vi "config-AUXI.vi"(11 "DO List":string[](array[string])) -> ()   [LabVIEW 2024]
uses:
  controls/type.aux.ctl
  <vilib>/Utility/miscctls.llb/LVPointTypeDef.ctl
  controls/typeEnv.ctl
  controls/UiProcHeader.ctl
  <vilib>/Utility/error.llb/Clear Errors.vi
  globals/globals-engine.vi
  <vilib>/Utility/libraryn.llb/Create Directory Recursive.vi
panel:
  in  "Cluster":T1={"Source"="Source ...", "SourceStatus"=FALSE, "Dest"="Auxiliary ...", "DestStatus"=FALSE, "Pulse"=0, "Period"=0, "Proc Name"=""} {"Period" format="Period [s]: %d"; "Pulse" format="Pulse [s]: %d"}
  in  "index":i8=1 min=1 max=10 step=1
  out "deleted path":path
  in  "Menu":cluster{"load":bool, "save":bool}
  in  "Aux Conf":T1[](array[typedef]) {"Period" format="Period [s]: %d"; "Pulse" format="Pulse [s]: %d"}
  in  "DataChanged?":bool=TRUE
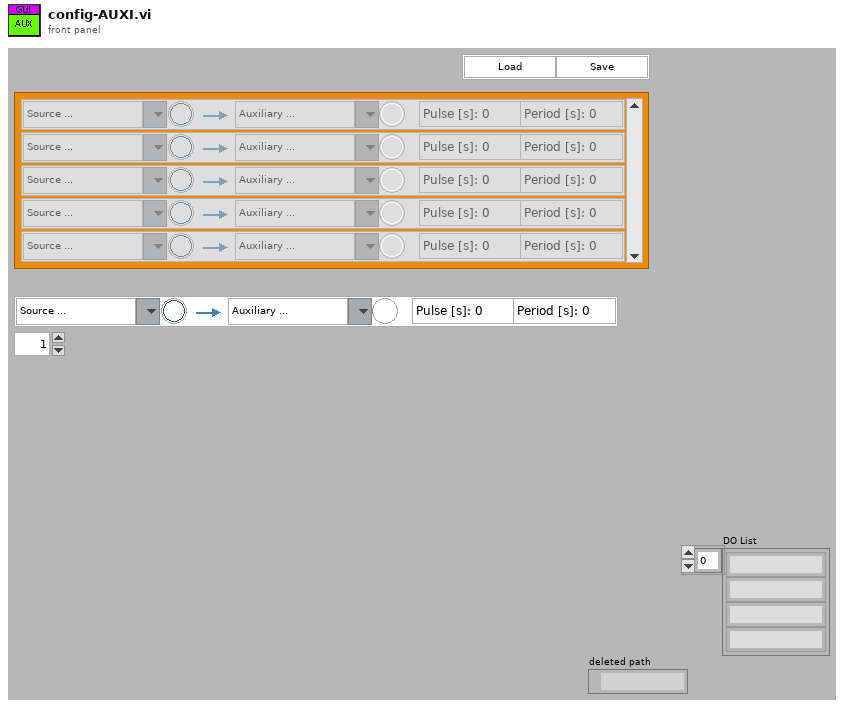
[diagram p1: front panel]
types:
  T1 = typedef "type.aux.ctl" = cluster{"Source":string, "SourceStatus":bool, "Dest":string, "DestStatus":bool, "Pulse":u16, "Period":u16, "Proc Name":string}
  T2 = typedef "typeEnv.ctl" = enum16{"ENV.PRODUCTION", "ENV.TEST.NO-HW", "ENV.TEST.SINGLE-01", "ENV.TEST.SINGLE-02", "ENV.TEST.SINGLE-02 AI 0", "ENV.TEST.SINGLE-03"}
  T3 = typedef "LVPointTypeDef.ctl" = cluster{"Horizontal":i16, "Vertical":i16}
  T4 = typedef "UiProcHeader.ctl" = cluster{"Procedure Name":string, "Running":bool, "tags":string}
  T5 = typedef "UiStepBuilder.ctl" = cluster{"Step Function":T6, "ParamString":string, "Step Label":string}
  T6 = typedef "type.step-builder.ctl" = enum16{"NO_OPERATION", "DELAY-JUMP", "DELAY", "JUMP", "COMPLETE", "SCHEDULER", "IRR-CHECK", "UNIT-CHECK", "UNIT-SAMPLE", "UNIT-DOSE", "LOG-REPORT", "LOG-MESSAGE", "IO-READ", "IO-READ-MANY", "IO-WRITE", "IO-COMPARE-OUT", "IO-COMPARE-IN", "PROC-START", "PROC-STOP", "PROC-LOAD", "PROC-IS-COMPLETED", "RECORD-MOVE", "GET-RH", "GET-UV", "GET-WD", "GET-WS", "OCS-CHECK", "OCS-RECORD"}
  T7 = enum32{"Invalid", "Standard", "Closed", "Hidden", "Minimized", "Maximized"}
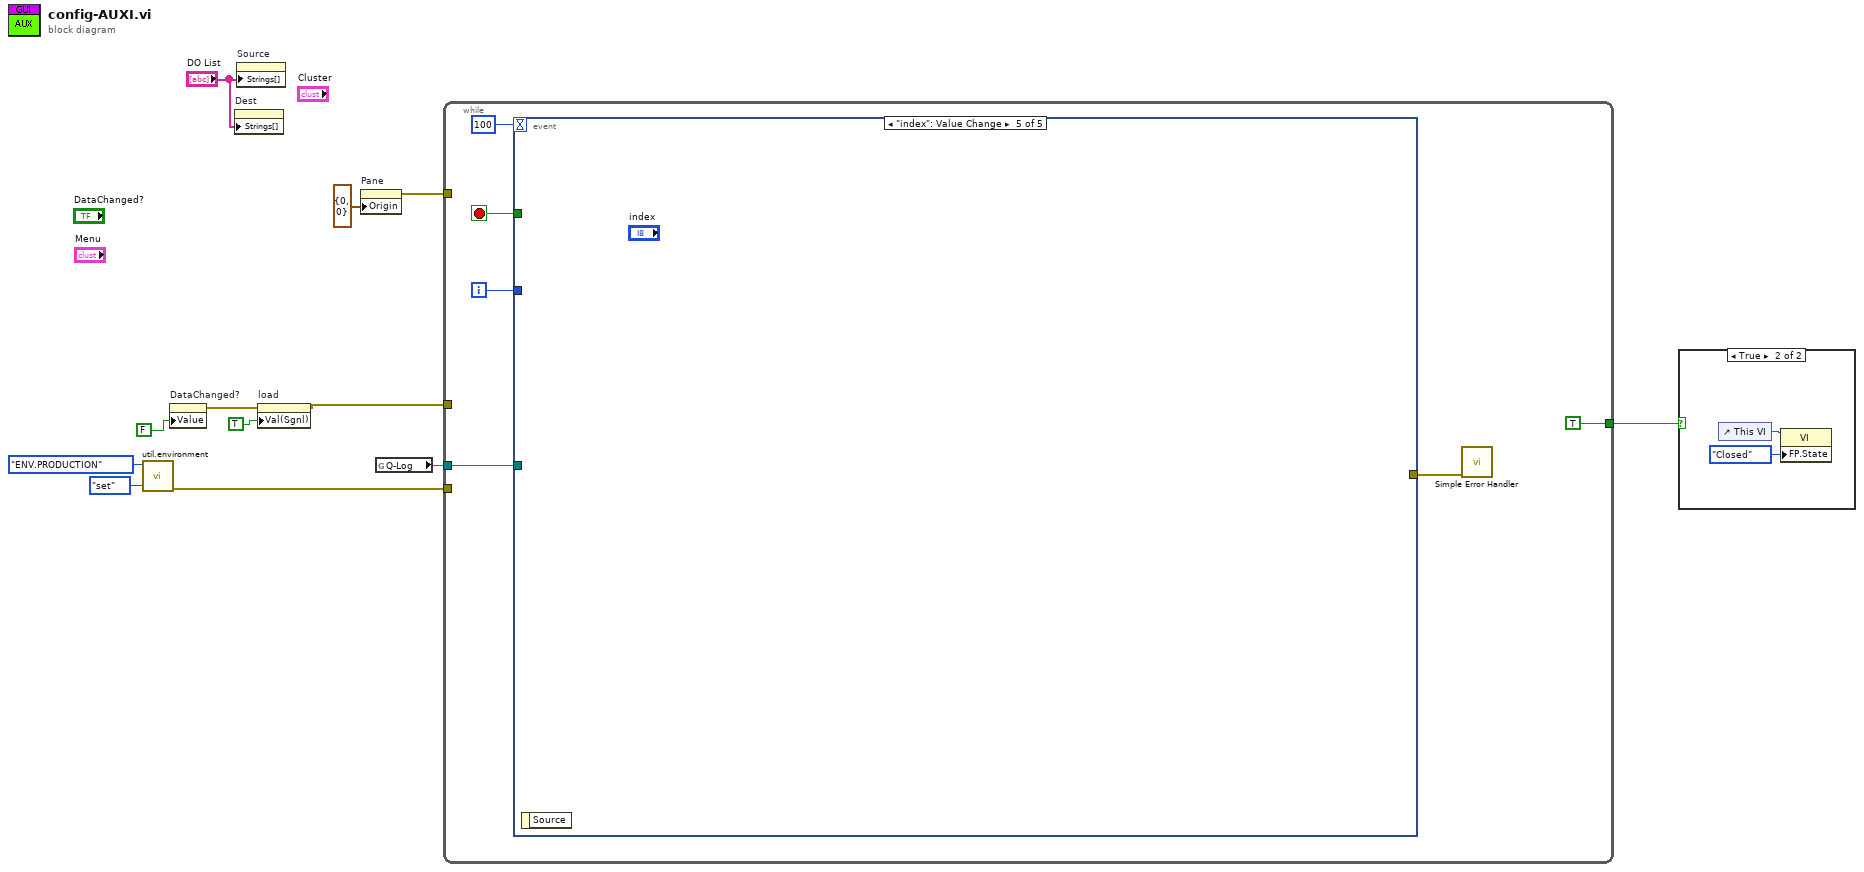
[diagram p0: block diagram]
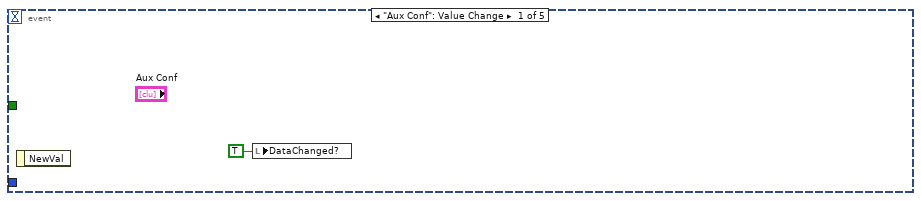
[diagram p3: hidden frame]
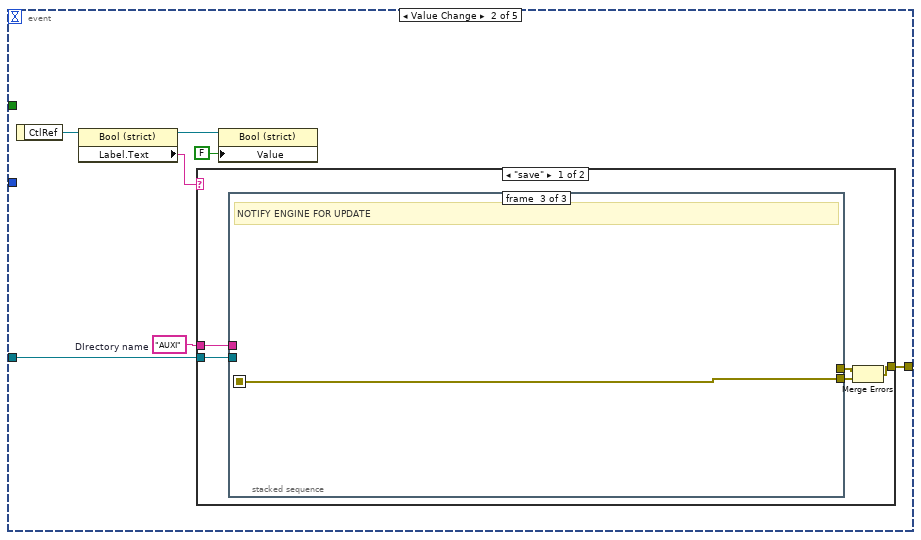
[diagram p4: hidden frame]
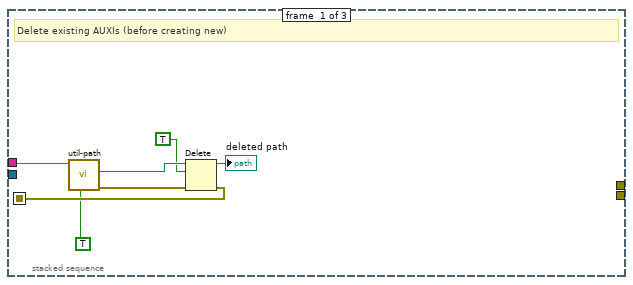
[diagram p5: hidden frame]
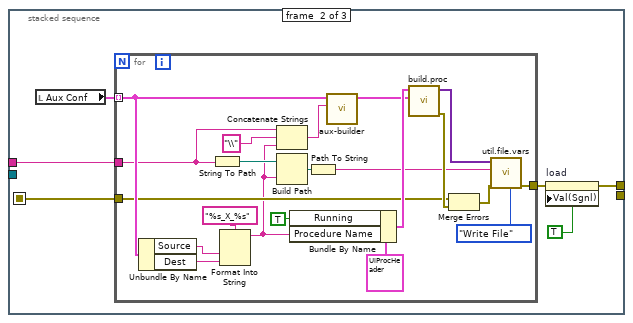
[diagram p6: hidden frame]
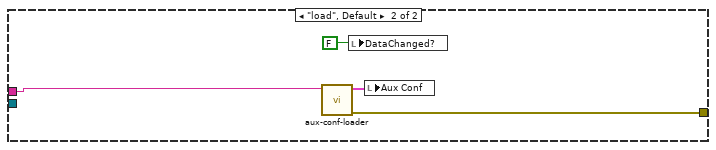
[diagram p7: hidden frame]
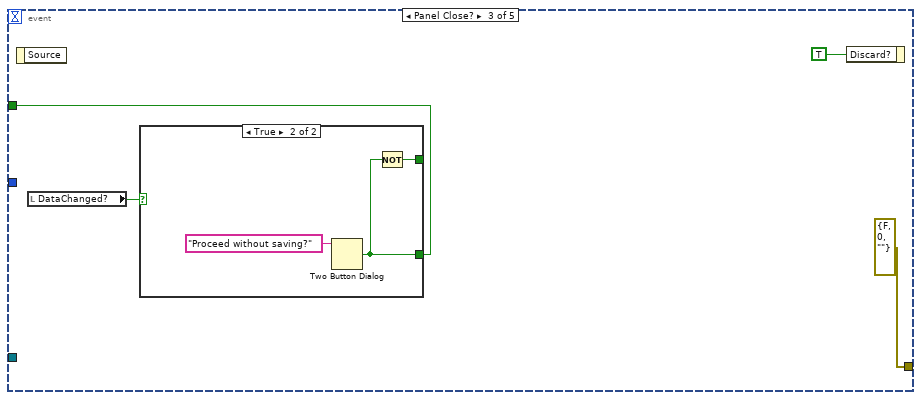
[diagram p8: hidden frame]
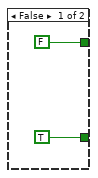
[diagram p9: hidden frame]
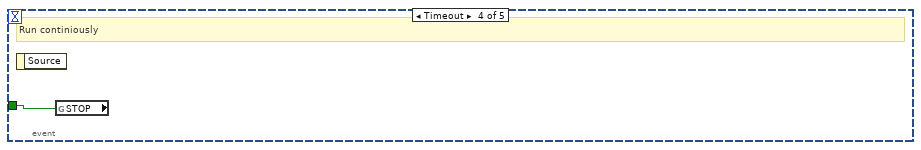
[diagram p10: hidden frame]
diagram:
  n1 = call "util.environment.vi"("Operation (Get)"=enum16{"get", "set"}."set" ("Operation"), "ENV in"=typeEnv."ENV.PRODUCTION") -> ("error out"=w10:errorcluster)  [unwired: 8 in, 1 out]
  n2 = property on="DataChanged?" class="Bool (strict)"("Value"=FALSE ("Value (Signaling)")) -> (error out=w3:errorcluster)  [unwired: 2 in, 1 out]
  n3 = property on="Dest" class="CmbBox"("Strings[]"="DO List") -> ()  [unwired: 2 in, 2 out]
  n4 = property on="Source" class="CmbBox"("Strings[]"="DO List") -> ()  [unwired: 2 in, 2 out]
  n5 = property on="load" class="Bool (strict)"(error in=w3, "Val(Sgnl)"=TRUE ("Value (Signaling)")) -> (error out=w6:errorcluster)  [unwired: 1 in, 1 out]
  n6 = property on="Pane" class="Pane"("Origin"=T3 {"Horizontal"=0, "Vertical"=0}) -> (error out=w12:errorcluster)  [unwired: 2 in, 1 out]
  n7 = global read "globals-engine.vi" "Q-Log"() -> (w1:refnum<queue>)
  n8 = while {
    tunnel: w12 -> [_]
    tunnel: w10 -> [_]
    tunnel: [TRUE] -> w7
    tunnel: w6 -> [_]
    tunnel: w1 -> [w13]
    i -> [w14]
    stop <- w18 stop-if-true
    n9 = event shown="[4] \"index\": Value Change" {
      selector: _ -> [_ _ _ _ _]
      dyn-events: _ -> [_ _ _ _ _]
      timeout: 100 ("Event TO") -> [_ _ _ _ _]
      tunnel: [_ _ w72 w80 _] -> w18
      tunnel: [_ w22 errorcluster {"status"=FALSE, "code"=0, "source"=""} ("error out") _ _] -> w15
      tunnel: w14 -> [_ _ _ _ _]
      tunnel: w13 -> [_ w20 _ _ _]
      event "Aux Conf": Value Change {
        n10 = event-data() -> ()  [unwired: 1 in, 1 out]
        n11 = local write "DataChanged?"(TRUE ("DataChanged?")) -> ()
      }
      event "Menu.load", "Menu.save": Value Change {
        w21 = "AUXI"  # DIrectory name
        n12 = event-data() -> ("CtlRef"=w26:refnum<vi>)  [unwired: 1 in]
        n13 = property class="Bool (strict)"(reference=w26) -> (reference out=w24:refnum<vi>, "Label.Text"=w25:string)  [unwired: 1 in, 1 out]
        n14 = case shown="\"save\"" w25 {
          tunnel: [w29 w68] -> w22
          tunnel: w21 -> [w30 w67]
          tunnel: w20 -> [w27 _]
          frame "save" {
            n15 = stacked-sequence {
              seq-local: [w35 _ _] -> [_ w40 w66]
              tunnel: [_ w41 _] -> w31
              tunnel: w30 -> [w33 w39 _]
              tunnel: [_ _ w66] -> w28
              tunnel: w27 -> [_ _ _]
              frame #0 {
                # "Delete existing AUXIs (before creating new)"
                n16 = call "util-path.vi"("Create Folders?(F)"=TRUE, "append path (ie. folder\\filename.*)"=w33) -> ("error out"=w37:errorcluster, "SelectedPath"=w38:path)  [unwired: 5 in, 3 out]
                n17 = Delete(path (use dialog)=w38, entire hierarchy (F)=TRUE, error in=w37) -> (deleted path=→"deleted path":path, error out=w35:errorcluster)  [unwired: 2 in, 1 out]
              }
              frame #1 {
                n18 = local read "Aux Conf"() -> (w43:T1[])
                n19 = for {
                  tunnel: [w58] -> w44
                  tunnel: w43 -> [w56] mode=indexing
                  tunnel: w40 -> [w49]
                  tunnel: w39 -> [w48]
                  n20 = Unbundle By Name(w56) -> ("Source"=w54:string, "Dest"=w53:string)
                  n21 = String To Path(string=w48) -> (path=w57:path)
                  n22 = Format Into String(format string="%s_X_%s", w54, w53) -> (resulting string=w46:string)  [unwired: 2 in, 1 out]
                  n23 = Concatenate Strings(w48, "\\" ("string"), w46) -> (w45:string)
                  n24 = Build Path(base path=w57, name or relative path=w46) -> (appended path=w52:path)
                  n25 = Bundle By Name(cluster=T4 {"Procedure Name"="MyProcExample", "Running"=TRUE, "tags"="MyProcExample"} ("Proc Head"), "Running"=TRUE, "Procedure Name"=w46) -> (w63:T4)
                  n26 = Path To String(path=w52) -> (string=w51:string)
                  n27 = call "aux-builder.vi"("Proc Name"=w45, "Cluster"=w56) -> ("AUXI Flow"=w59:T5[])  [unwired: 9 in]
                  n28 = call "build.proc.vi"("Flow"=w59, "Proc Head"=w63) -> ("error out"=w65:errorcluster, "Instructions"=w64:variant[])  [unwired: 8 in]
                  n29 = Merge Errors(w49, w65) -> (w50:errorcluster)
                  n30 = call "util.file.vars.vi"("Operation(Read)"=enum16{"Read File", "Write File"}."Write File", "error in"=w50, "Proc Name(open dialog if empty)"=w51, "Vars[] in"=w64) -> ("error out"=w58:errorcluster)  [unwired: 3 in, 4 out]
                }
                n31 = property on="load" class="Bool (strict)"(error in=w44, "Val(Sgnl)"=TRUE ("Value (Signaling)")) -> (error out=w41:errorcluster)  [unwired: 1 in, 1 out]
              }
              frame #2 {
                # "NOTIFY ENGINE FOR UPDATE"
              }
            }
            n32 = Merge Errors(w31, w28) -> (w29:errorcluster)
          }
          frame "load", Default {
            n33 = call "aux-conf-loader.vi"("DIrectory (AUXI)"=w67) -> ("error out"=w68:errorcluster, "Array"=w69:T1[])  [unwired: 9 in]
            n34 = local write "DataChanged?"(FALSE ("Value (Signaling)")) -> ()
            n35 = local write "Aux Conf"(w69) -> ()
          }
        }
        n36 = property class="Bool (strict)"(reference=w24, "Value"=FALSE) -> ()  [unwired: 1 in, 2 out]
      }
      event Panel Close? {
        n37 = event-data() -> ()  [unwired: 1 in, 1 out]
        n38 = local read "DataChanged?"() -> (w73:bool)
        n39 = case shown="True" w73 {
          tunnel: [FALSE ("T button?") w77] -> _
          tunnel: [TRUE ("T button?") w78] -> w72
          frame False {
          }
          frame True {
            n40 = Two Button Dialog(message="Proceed without saving?") -> (T button?=w78:bool)  [unwired: 2 in]
            n41 = Not(x=w78) -> (.not. x?=w77:bool)
          }
        }
        n42 = event-data("Discard?"=TRUE) -> ()  [unwired: 1 in, 1 out]
      }
      event Timeout {
        # "Run continiously"
        n43 = event-data() -> ()  [unwired: 1 in, 1 out]
        n44 = global read "globals-engine.vi" "STOP"() -> (w80:bool)
      }
      event "index": Value Change {
        n45 = event-data() -> ()  [unwired: 1 in, 1 out]
      }
    }
    n46 = call <vilib>:"Simple Error Handler.vi"("error in (no error)"=w15) -> ()  [unwired: 4 in, 5 out]
  }
  n47 = case shown="True" w7 {
    frame False {
    }
    frame True {
      n48 = control-ref of="This VI"() -> (w82:refnum<vi>)
      n49 = property class="VI"(reference=w82, "FP.State"=T7."Closed" ("Front Panel Window:State")) -> ()  [unwired: 1 in, 2 out]
    }
  }
